vi "Motor_PIDFilter.vi"(6 "Initialize (F)":bool, 7 "Softload? (T)":bool=TRUE, 8 "error in (no error)":errorcluster, 9 "PID cmd in":dbl[](array[numeric])=[0.0] format="%.2f", 10 "FF cmd in":dbl[](array[numeric])=[0.0] format="%.2f", 11 "Motors_New in":refnum<class "MotorControl.lvclass">) -> (0 "error out":errorcluster, 1 "Filtered PID":dbl[](array[numeric]) format="%.2f", 2 "Filtered PID + FF":dbl[](array[numeric]) format="%.2f", 3 "Motors_New out":refnum<class "MotorControl.lvclass">)   [LabVIEW 2015, in "MotorControl.lvclass"]
uses:
  MotorControl.lvclass
  MotorControl.lvclass/MotorControl.ctl
  <vilib>/addons/control/pid/pid.llb/PID Output Rate Limiter (DBL Array).vi
  <vilib>/addons/control/pid/NI_PID_pid.lvlib
panel:
  out "Output Rate (V/min)":dbl[](array[numeric])
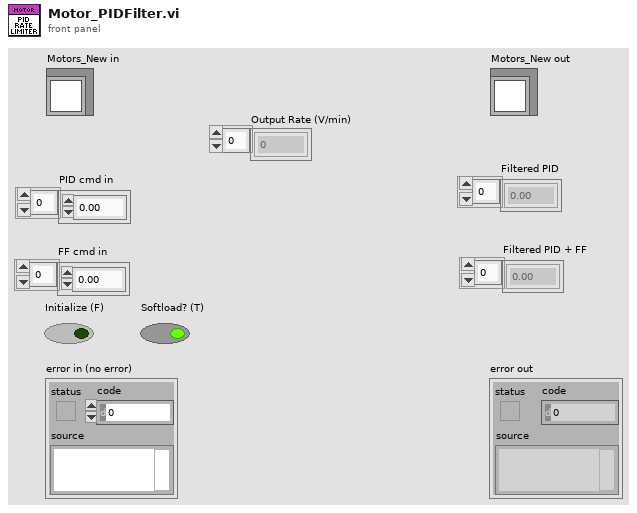
[diagram p1: front panel]
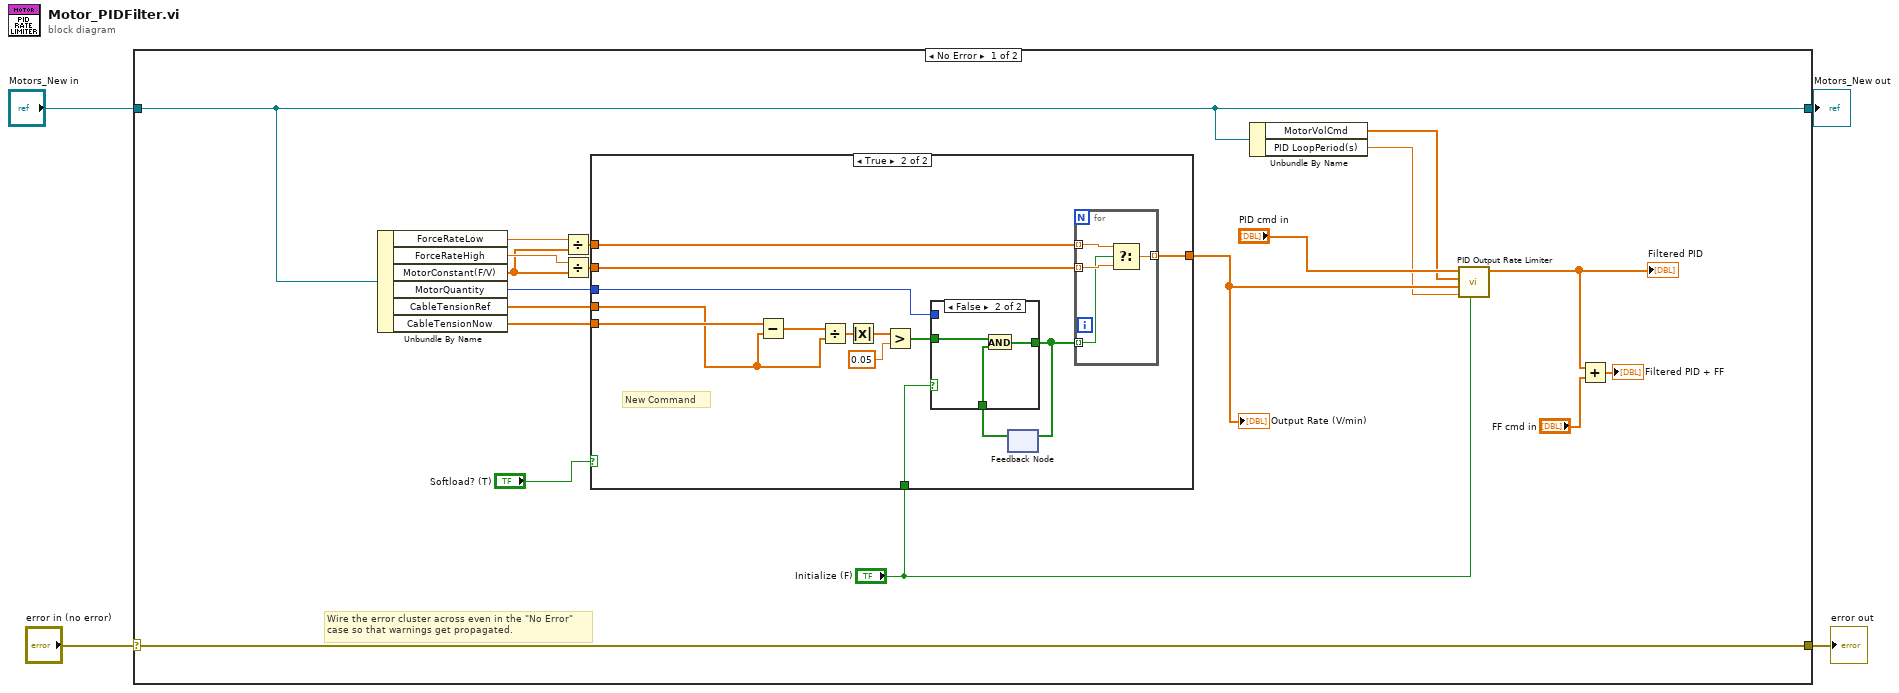
[diagram p0: block diagram]
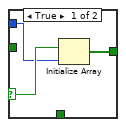
[diagram p3: hidden frame]
diagram:
  n1 = case shown="No Error" "error in (no error)" {
    selector: "error in (no error)" -> [w23 w50]
    tunnel: [w23 w50] -> w3
    tunnel: [w11 w49] -> w1
    tunnel: "Motors_New in" -> [w11 w49]
    frame No Error {
      # "Wire the error cluster across even in the \"No Error\"\ncase so that warnings get propagated."
      n2 = Unbundle By Name(w11) -> ("ForceRateLow"=w22:dbl, "ForceRateHigh"=w21:dbl, "MotorConstant(F/V)"=w20:dbl[], "MotorQuantity"=w17:i32, "CableTensionRef"=w14:dbl[], "CableTensionNow"=w15:dbl[])
      n3 = Divide(x=w22, y=w20) -> (x/y=w19:dbl[])
      n4 = Divide(x=w21, y=w20) -> (x/y=w18:dbl[])
      n5 = case shown="True" "Softload? (T)" {
        tunnel: w19 -> [_ w38]
        tunnel: w18 -> [w24 w37]
        tunnel: w17 -> [_ w30]
        tunnel: [w24 w29] -> w13
        tunnel: w15 -> [_ w28]
        tunnel: w14 -> [_ w27]
        tunnel: "Initialize (F)" -> [_ w25]
        frame False {
        }
        frame True {
          # "New Command"
          n6 = Subtract(x=w28, y=w27) -> (x-y=w35:dbl[])
          n7 = Divide(x=w35, y=w27) -> (x/y=w36:dbl[])
          n8 = Absolute Value(x=w36) -> (abs(x)=w34:dbl[])
          n9 = Greater?(x=w34, y=0.05) -> (0:w32:bool[])
          n10 = feedback #1() -> (w26:bool[])  [unwired: 1 in]
          n11 = case shown="False" w25 {
            selector: w25 -> [w41 _]
            tunnel: w32 -> [_ w43]
            tunnel: [w39 w44] -> w31
            tunnel: w30 -> [w40 _]
            tunnel: w26 -> [_ w42]
            frame True {
              n12 = Initialize Array(w41, w40) -> (w39:bool[])
            }
            frame False {
              n13 = And(x=w43, y=w42) -> (x .and. y?=w44:bool[])
            }
          }
          n14 = feedback-in #1(w31) -> ()
          n15 = for {
            tunnel: w38 -> [w48] mode=indexing
            tunnel: w37 -> [w47] mode=indexing
            tunnel: [w46] -> w29 mode=indexing
            tunnel: w31 -> [w45] mode=indexing
            n16 = Select(t=w48, s=w45, f=w47) -> (s? t:f=w46:dbl)
          }
        }
      }
      "Output Rate (V/min)" <- w13
      n17 = Unbundle By Name(w11) -> ("MotorVolCmd"=w10:dbl[], "PID LoopPeriod(s)"=w9:dbl)
      n18 = call-poly <vilib>:"PID Output Rate Limiter.vi"("reinitialize? (F)"="Initialize (F)", "dt (s)"=w9, "output rate (EGU/min)"=w13, "initial output"=w10, "input (controller output)"="PID cmd in") -> ("output"=w6:dbl[])  [unwired: 3 in, 1 out]
      "Filtered PID" <- w6
      n19 = Add(x=w6, y="FF cmd in") -> (x+y=→"Filtered PID + FF":dbl[])
    }
    frame Error {
    }
  }
  "error out" <- w3
  "Motors_New out" <- w1
